vi "Read Coords.vi"(8 "error in (no error)":errorcluster, 11 "ControlDropMsg in":refnum<class "ControlDropMsg.lvclass">) -> (0 "error out":errorcluster, 2 "Coords":T1, 3 "ControlDropMsg out":refnum<class "ControlDropMsg.lvclass">)   [LabVIEW 2018, in "MVA Framework.lvlib" / "ActorEvents.lvlib" / "ControlDropMsg.lvclass"]
uses:
  ControlDropMsg.lvclass
  <vilib>/Utility/miscctls.llb/LVPoint32TypeDef.ctl
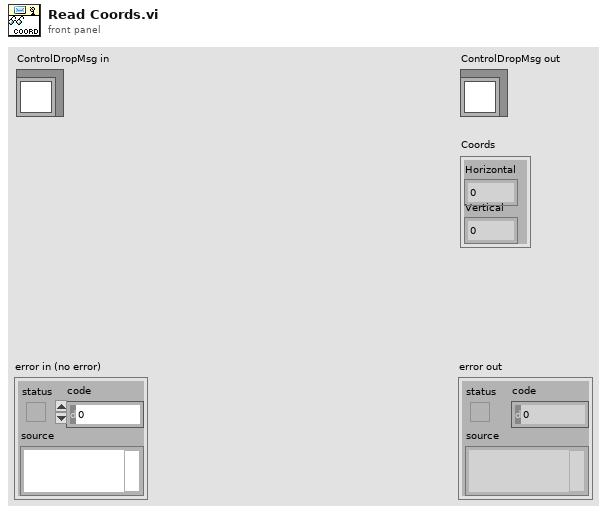
[diagram p1: front panel]
types:
  T1 = typedef "LVPoint32TypeDef.ctl" = cluster{"Horizontal":i32, "Vertical":i32}
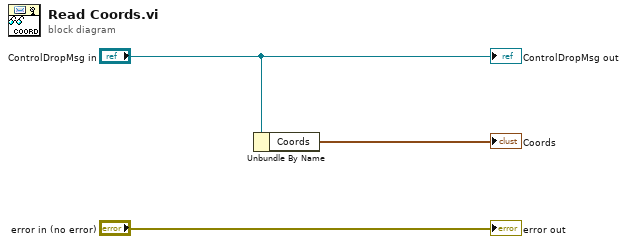
[diagram p0: block diagram]
diagram:
  n1 = Unbundle By Name("ControlDropMsg in") -> ("Coords"=→"Coords":T1)
  "error out" <- "error in (no error)"
  "ControlDropMsg out" <- "ControlDropMsg in"
